vi "Destroy.vi"(8 "error in (no error)":errorcluster, 11 "Synchronous Request Callback In":refnum<class "Synchronous Request Callback.lvclass">) -> (0 "error out":errorcluster)   [LabVIEW 2020, in "Synchronous Request Callback.lvclass"]
uses:
  Synchronous Request Callback.lvclass
  Synchronous Request Callback.lvclass/Synchronous Request Callback.ctl
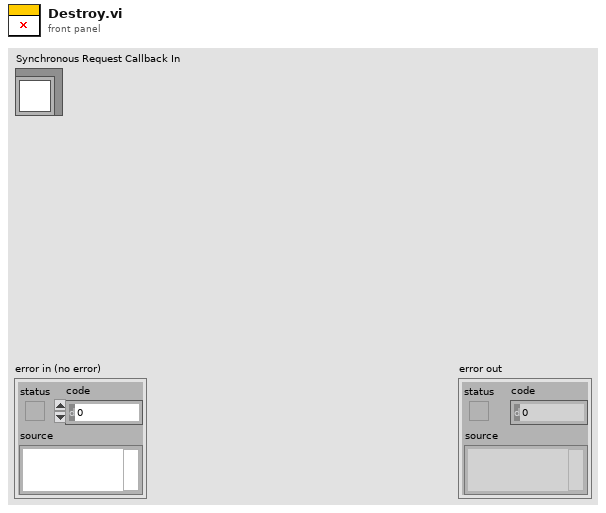
[diagram p1: front panel]
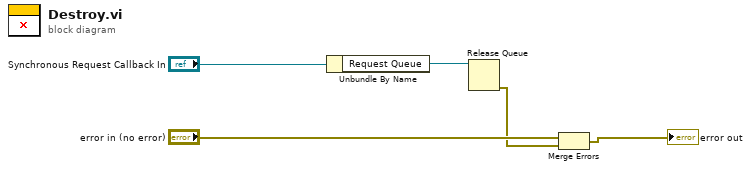
[diagram p0: block diagram]
diagram:
  n1 = Unbundle By Name("Synchronous Request Callback In") -> ("Request Queue"=w3:refnum<queue>)
  n2 = Release Queue(queue=w3) -> (error out=w1:errorcluster)  [unwired: 2 in, 2 out]
  n3 = Merge Errors("error in (no error)", w1) -> (→"error out":errorcluster)
